vi "DIO Example (A).vi"() -> ()   [LabVIEW 2011]
uses:
  C:/Program Files/Metrohm Autolab/Autolab SDK 1.10/EcoChemie.Autolab.Sdk.dll
  EcoChemie.Autolab.Sdk.dll
panel:
  out "DIO Status P2 R":bool[](array[boolean])
  in  "DIO Status P2 W":bool[](array[boolean])
  in  "Port P2":i32(ring) items=["Port_A", "Port_B", "Port_C"]
  in  "P2 Direction":enum16{"Input(read)", "Output(write)"}(ring)
  out "DIO Status P1 R":bool[](array[boolean])
  in  "Port P1":i32(ring) items=["Port_A", "Port_B", "Port_C"]
  in  "P1 Direction":enum16{"Input(read)", "Output(write)"}(ring)
  in  "DIO Status P1 W":bool[](array[boolean])
  out "error out":errorcluster
  in  "stop":bool
  out "IsConnected":bool
  in  "Hardware Setup File":path
  in  "Embedded Exe File":path
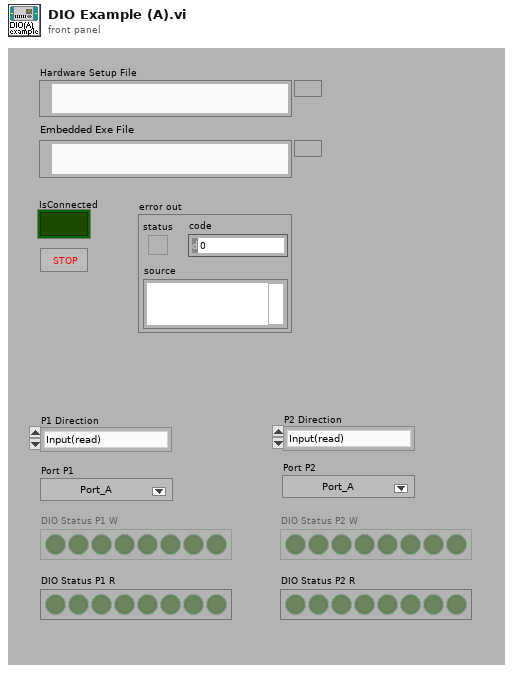
[diagram p1: front panel]
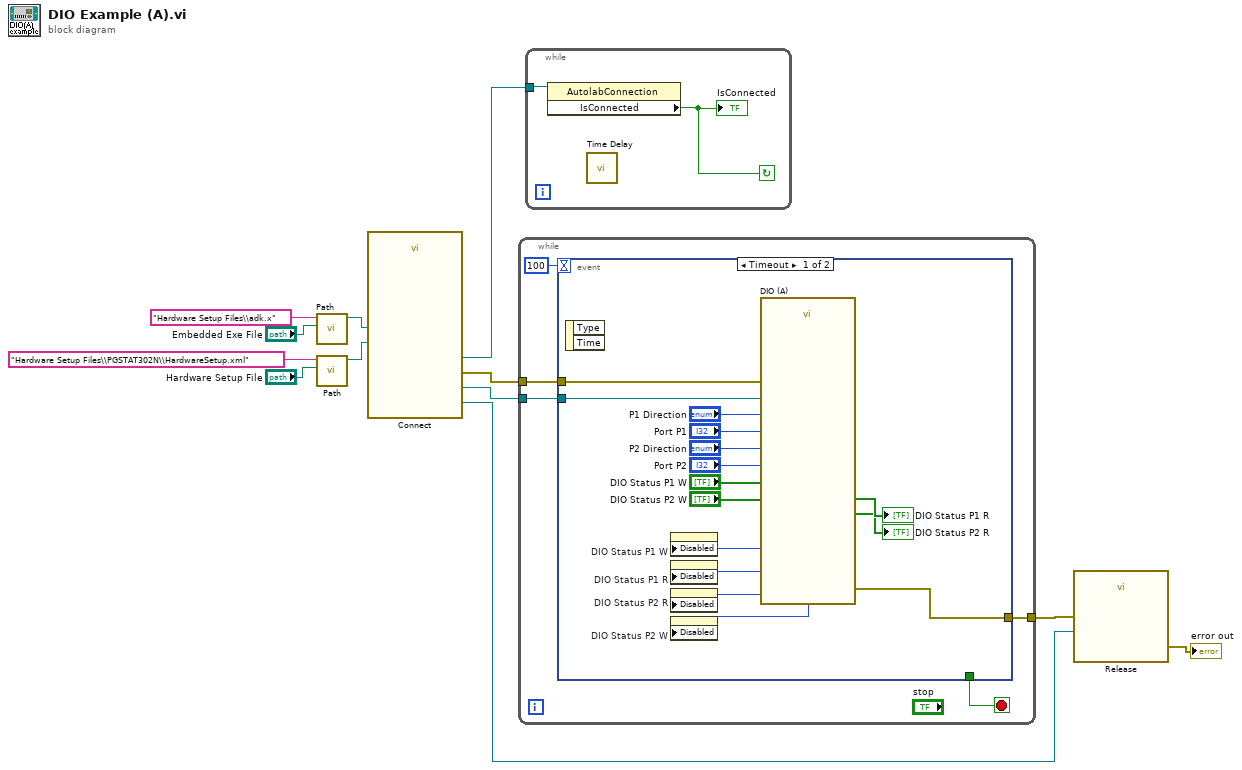
[diagram p0: block diagram]
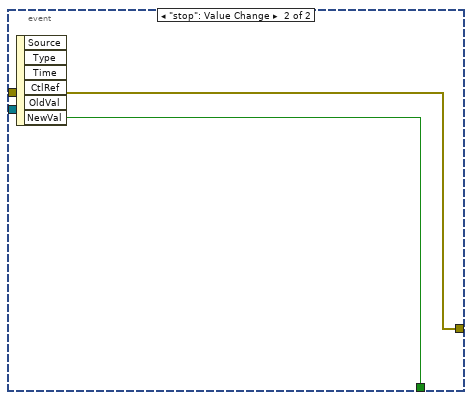
[diagram p2: hidden frame]
diagram:
  n1 = call "Path.vi"("File"="Embedded Exe File", "name or relative path"="Hardware Setup Files\\adk.x") -> ("appended path"=w4:path)  [unwired: 9 in]
  n2 = call "Path.vi"("File"="Hardware Setup File", "name or relative path"="Hardware Setup Files\\PGSTAT302N\\HardwareSetup.xml") -> ("appended path"=w3:path)  [unwired: 9 in]
  n3 = call "Connect.vi"("Embedded Exe File"=w4, "Hardware Setup File"=w3) -> ("Dio"=w9:refnum<k24>, "AutolabConnection"=w7:refnum<k24>, "instrument"=w10:refnum<k24>, "error out"=w8:errorcluster)  [unwired: 6 in, 4 out]
  n4 = while {
    tunnel: [w17] -> w11
    tunnel: w9 -> [w16]
    tunnel: w8 -> [w15]
    stop <- w13 stop-if-true
    n5 = event shown="[0] Timeout" {
      selector: _ -> [_ _]
      dyn-events: _ -> [_ _]
      timeout: 100 -> [_ _]
      tunnel: [w20 w33] -> w17
      tunnel: w16 -> [w19 _]
      tunnel: w15 -> [w18 w33]
      tunnel: [_ w34] -> w13
      event Timeout {
        n6 = event-data() -> ()  [unwired: 1 in, 2 out]
        n7 = call "DIO (A).vi"("Dio"=w19, "DIO Status P1 W"="DIO Status P1 W", "DIO Status P2 W"="DIO Status P2 W", "error in (no error)"=w18, "Port P1"="Port P1", "Port P2"="Port P2", "P1 Direction"="P1 Direction", "P2 Direction"="P2 Direction") -> ("Disable P1 W"=w24:u8, "Disable P2 W"=w21:u8, "DIO Status P1 R"=→"DIO Status P1 R":bool[], "Disable P1 R"=w23:u8, "DIO Status P2 R"=→"DIO Status P2 R":bool[], "Disable P2 R"=w22:u8, "error out"=w20:errorcluster)  [unwired: 5 in]
        n8 = property on="DIO Status P1 W" class="Arr (strict)"("Disabled"=w24) -> ()  [unwired: 2 in, 2 out]
        n9 = property on="DIO Status P1 R" class="Arr (strict)"("Disabled"=w23) -> ()  [unwired: 2 in, 2 out]
        n10 = property on="DIO Status P2 R" class="Arr (strict)"("Disabled"=w22) -> ()  [unwired: 2 in, 2 out]
        n11 = property on="DIO Status P2 W" class="Arr (strict)"("Disabled"=w21) -> ()  [unwired: 2 in, 2 out]
      }
      event "stop": Value Change {
        n12 = event-data() -> ("NewVal"=w34:bool)  [unwired: 1 in, 5 out]
      }
    }
  }
  n13 = while {
    tunnel: w7 -> [w36]
    stop <- w35 continue-if-true
    n14 = property class="AutolabConnection"(reference=w36) -> ("IsConnected"=w35:bool)  [unwired: 1 in, 2 out]
    "IsConnected" <- w35
    n15 = call "Time Delay"() -> ()  [unwired: 11 in, 1 out]
  }
  n16 = call "Release.vi"("error in (no error)"=w11, "Instrument"=w10) -> ("error out"=→"error out":errorcluster)  [unwired: 9 in]
